vi "Destroy Module Semaphore Reference.vi"(8 "error in":errorcluster, 11 "semaphore":T1) -> (0 "error out":errorcluster)   [LabVIEW 2019, in "Filepath Editor.lvlib"]
doc: "Destroy the module semaphore reference.\n_____\nBased on DQMH Project Template 6.1.0.94."
uses:
  Filepath Editor.lvlib
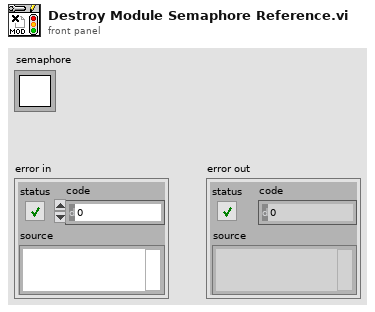
[diagram p1: front panel]
types:
  T1 = typedef "Semaphore RefNum" = refnum<k1>
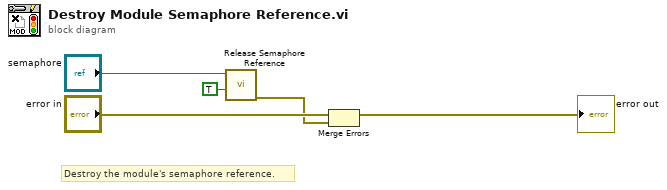
[diagram p0: block diagram]
diagram:
  # "Destroy the module's semaphore reference."
  n1 = call <vilib>:"Release Semaphore Reference.vi"("force destroy? (F)"=TRUE, "semaphore"="semaphore") -> ("error out"=w3:errorcluster)  [unwired: 8 in, 1 out]
  n2 = Merge Errors("error in", w3) -> (→"error out":errorcluster)
